vi "Debug Exercise (Sub).vi"(1 "Number":dbl format="%.2f") -> (0 "Final Result":dbl format="%.2f")   [LabVIEW 2011]
doc: "This VI is a subVI for an exercise in the LabVIEW Core I course.\n\nThis exercise is used to demonstrate the use of different debugging tools. First, fix the broken run arrow and then use the different debugging tools to see how they work."
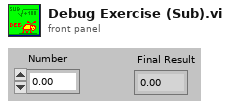
[diagram p1: front panel]
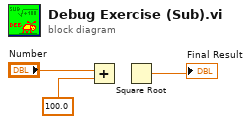
[diagram p0: block diagram]
diagram:
  n1 = Add(x="Number", y=100.0) -> ()  [unwired: 1 out]
  n2 = Square Root() -> (sqrt(x)=→"Final Result":dbl)  [unwired: 1 in]
